vi "main.vi"() -> ()   [LabVIEW 2011]
uses:
  Controls/Open Button.ctl
  Controls/Add2Plot Button.ctl
  Controls/Save Button.ctl
  Controls/Clear Button.ctl
  Controls/Export Button.ctl
  Controls/DAQ Type.ctl
  Controls/Run Button.ctl
  Controls/Stop Button.ctl
  Controls/Progress Bar.ctl
  Controls/Display Mode.ctl
  Controls/User Event Control.ctl
  Controls/User Event Action.ctl
  Controls/User Interface Action.ctl
  Controls/TDMS File Handling.ctl
  Modules/Menu/Menu Action.ctl
  Modules/File/TDMS/TDMS.lvclass
  Functional Global Data/Run Data.ctl
  <vilib>/event_ctls.llb/eventvkey.ctl
  Functional Global Data/Analysis Data.ctl
  Controls/Plot Parameters.ctl
  Functional Global Data/Status Bar.ctl
  Functional Global Data/Globals.ctl
  <vilib>/Utility/error.llb/DialogType.ctl
  Error Handling/Error Module Action.ctl
  <vilib>/Utility/file.llb/Write To Spreadsheet File (DBL).vi
  <vilib>/Analysis/NI_AALBase.lvlib
panel:
  in  "Stop Button":T1
  in  "start DAQ":T2
  in  "Experiment Type":T3
  in  "Open Button":T4
  in  "tab control":enum32{"Data", "Analysis"}(tab)
  in  "Display Mode":T5
  in  "Export History Button":T6
  in  "Run parameters":i32[](listbox)
  in  "Add History 2 Plot Button":T7
  in  "Add Spectrum 2 Plot Button":T7
  out "Notes":string
  out "Run":dbl[][](graph)
  out "Time":i32 caption="Time (s)"
  in  "Sample Channel Number":u32(slide)=1 caption="Sample Number" min=1 max=13 scale=1.0..13.0
  in  "Run Number":u16 caption="Run" min=1 max=1
  out "Sample":cluster{"xo":i32, "dx":i32, dbl[][]}(graph)
  in  "Sample Parameters":i32[](listbox)
  out "Analysis Plot Average":dbl caption="Average"
  in  "Save Concentration Plot Button":T8
  out "Concentration Plot":cluster{dbl[], dbl[]}(graph) caption="concentration VS IMS peak height"
  in  "Clear Plot Button":T9
  in  "Save Plot Button":T8
  out "Analysis Sample Plot":dbl[][](graph)
  out "Progress Bar":T10 scale=0.0..100.0
  out "Status Bar":string="MFC ();"
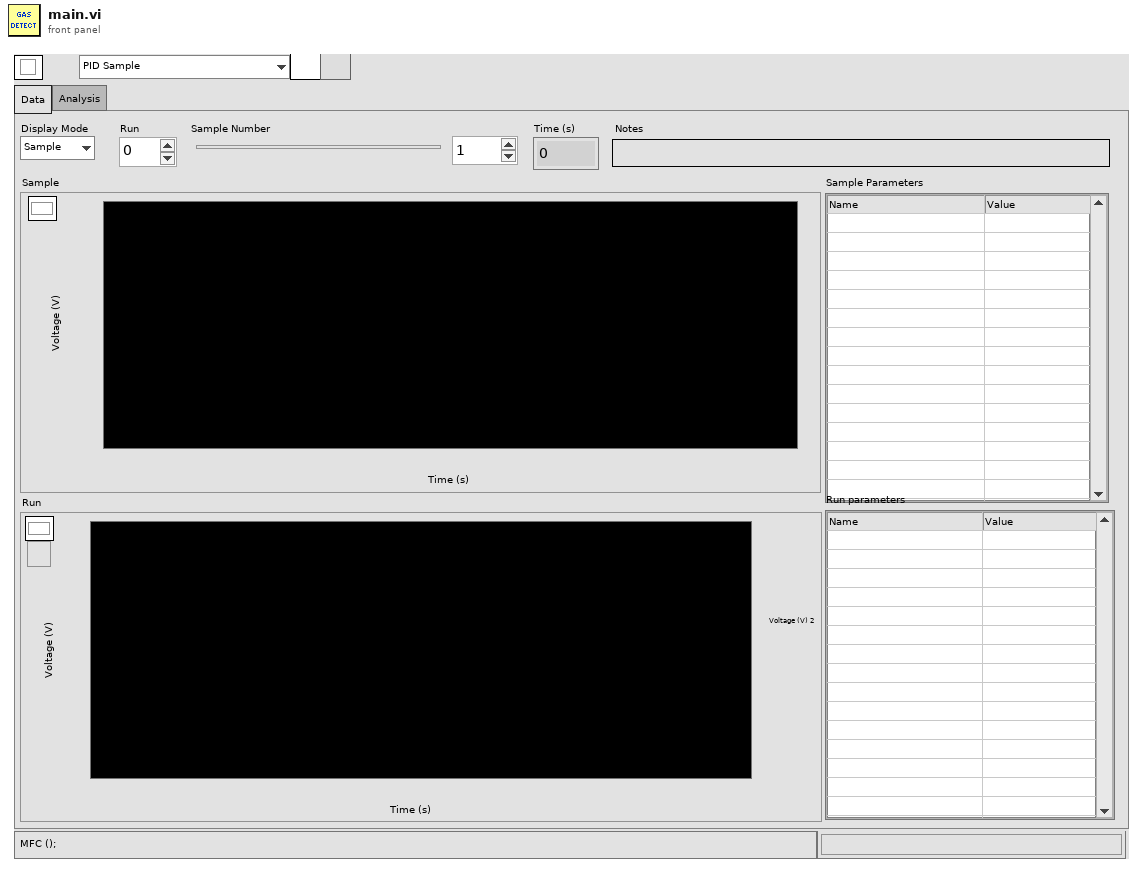
[diagram p1: front panel]
types:
  T1 = typedef "Stop Button.ctl" = bool
  T2 = typedef "Run Button.ctl" = bool
  T3 = typedef "DAQ Type.ctl" = enum16{"PID Sample", "PID with PS Challenge", "PID with MFC Challenge", "Multimeter Sample", "Multimeter with MFC Challenge"}
  T4 = typedef "Open Button.ctl" = bool
  T5 = typedef "Display Mode.ctl" = enum16{"Sample", "Run"}
  T6 = typedef "Export Button.ctl" = bool
  T7 = typedef "Add2Plot Button.ctl" = bool
  T8 = typedef "Save Button.ctl" = bool
  T9 = typedef "Clear Button.ctl" = bool
  T10 = typedef "Progress Bar.ctl" = u8
  T11 = typedef "Class Objects.ctl" = cluster{"configuration":refnum<class "Configuration.lvclass">, "TDMS":refnum<class "TDMS.lvclass">[], "Power Supply":refnum<class "Power Supply.lvclass">, "Mass Flow Controller":refnum<class "Mass Flow Controller.lvclass">, "Valve Controller":refnum<class "Valve Controller.lvclass">, "Multimeter":refnum<class "Multimeter.lvclass">, "Vapour Generator":refnum<class "Vapour Generator.lvclass">, "PIDs":refnum<class "PID.lvclass">[]}
  T12 = typedef "User Event Control.ctl" = cluster{"action":T13, "data":variant}
  T13 = typedef "User Event Action.ctl" = enum16{"Program Initialization", "Device Connections", "Device Settings", "Options", "DAQ Init", "PID Sample Test", "PID with PS Challenge", "PID with MFC Challenge", "Multimeter Sample Test", "Multimeter with MFC Challenge", "DAQ Stop", "Open Data File", "View Data File", "Change Display Mode", "Load INL PID Run Data", "Load Baseline-Mocon PID Data", "Load Multimeter Data", "Set Channel Sample", "Key Down", "Add Spectrum to Plot", "Add History to Plot", "Export History to Excel", "Clear Plots", "Save Plot", "Save Spectral Variable", "History Cursor Release", "Analysis Plot Cursor Release", "Program Deinitialization"}
  T14 = typedef "Menu Action.ctl" = enum16{"Initialize", "Insert Item", "Remove Item", "Set Checked Item", "Get Checked Item", "Get Item Index", "Item Present?", "Stop"}
  T15 = typedef "Globals.ctl" = enum16{"Initialize", "Get DAQ Params", "Get Data Display Params", "Set DAQ Params", "Set Data Display Params"}
  T16 = typedef "User Interface Action.ctl" = enum16{"Initialize", "Data Acquisition Disable", "Data View Disable", "Sample Set", "Sample Set 2D Data", "Sample Set x0 & dx", "Sample Add", "Sample Set Cursor", "Sample Set Offset & Multiplier", "Sample Set Axis Labels", "Sample Parameters Disabled", "Sample Parameters Update", "Run Update", "Run Set Offset & Multiplier", "Run Set Axis Labels", "Run Set Cursor", "Run Set Disabled", "Run Parameters Update", "Run Parameters Disabled", "Run Number Set", "Run Number Set Range", "Run Number Set Disabled", "Sample Number Set", "Sample Number Set Range", "Notes Set Value", "Update Plot", "Set Plot Parameters", "Update Concentration Plot", "Time Set", "Clear DAQ Display", "Clear Analysis Display", "Status Bar Set", "Progress Bar Set", "Display Mode Set", "Experiment Type Set", "Analysis Plot Average Set", "Stop"}
  T17 = typedef "Error Module Action.ctl" = enum16{"Initialize", "Handle Errors", "Report Errors"}
  T18 = typedef "Data Acquisition Parameters.ctl" = cluster{"Experiment Type":T3, "Experiment Name":string, "Operator Name":string, "Notes":string, "TDMS File Path":path, "Data Acquisition State":bool, "PID Voltage Sweep":T19, "MFC Challenge Profile - Heaviside Step":T20, "MFC Challenge Profile":T21, "MFC Challenge Profile - Staircase":T22}
  T19 = typedef "PID Voltage Seep Settings.ctl" = cluster{"Voltage Step (V)":dbl, "Voltage Range (V)":cluster{u16, u16}, "Time Step (s)":dbl, "Voltage Step Direction":enum16{"High 2 Low", "Low 2 High"}}
  T20 = typedef "MFC Challenge Profile - Heaviside Step.ctl" = cluster{"Valve Open Duration":u16, "MFC Flow Rate":dbl, "Valve Open Repeats":u16, "Valve Open Start":u16}
  T21 = typedef "MFC Challen Profile Type.ctl" = enum16{"Heaviside", "Staircase"}
  T22 = typedef "MFC Challenge Profile - Staircase.ctl" = cluster{"Step Time Duration":u16, "Step Flow Rate":dbl, "Steps":u16, "Valve Open Start":u16, "Recovery":bool, "Repeats":u16}
  T23 = typedef "eventvkey.ctl" = enum16{"ASCII", "Enter", "Return", "Shift", "Ctrl", "Alt", "Cmd", "Opt", "Caps", "NumLock", "Clear", "Break", "Up", "Down", "Left", "Right", "Insert", "Delete", "Home", "End", "PageUp", "PageDown", "Escape", "Help", "Pause", "ScrollLock", "F1", "F2", "F3", "F4", "F5", "F6", "F7", "F8", "F9", "F10", "F11", "F12", "F13", "F14", "F15", "F16", "F17", "F18", "F19", "F20", "F21", "F22", "F23", "F24", "Play", "VolumeUp", "VolumeDown", "Mute", "Two Byte Char"}
  T24 = typedef "DialogType.ctl" = u16
  T25 = typedef "TDMS File Handling.ctl" = enum16{"Add TDMS File", "Get Active TDMS File", "Set Active TDMS File", "Set Active TDMS File Index"}
  T26 = typedef "Run Data.ctl" = enum16{"Initialize", "Add Sample Channel", "Set Run", "Get Number of Runs", "Set Run Params", "Get Spectrum", "Get Run Params", "Get Sample Params", "Get History", "Get Averaged History", "Get Run Param Names", "Set Run Param Names", "Get Sample Param Names", "Set Sample Param Names", "Get MFC Flow Rate Challenge Profile", "Get History Average"}
  T27 = typedef "imagedata.ctl" = cluster{"image type":i32, "image depth":i32, "image":u8[], "mask":u8[], "colors":u32[], "Rectangle":cluster{"left":i16, "top":i16, "right":i16, "bottom":i16}}
  T28 = enum8{"Enabled", "Disabled", "Disabled and Grayed Out"}
  T29 = typedef "Analysis Data.ctl" = enum16{"Initialize", "Add Plot", "Get Plots"}
  T30 = typedef "Plot Parameters.ctl" = cluster{"line style":enum16{"0", "1", "2", "3", "4"}, "line width":enum16{"0", "1", "2", "3", "4", "5"}, "plot color":u32}
  T31 = typedef "Status Bar.ctl" = enum16{"Insert Into Status Bar", "Get Status Bar", "Initialize"}
  T32 = enum16{"PID Sample", "PID with PS Challenge", "PID with MFC Challenge", "Multimeter Sample", "Multimeter with MFC Challenge"}
  T33 = typedef "User Interface Control.ctl" = cluster{"action":T16, "data1":variant, "data2":variant}
  T34 = typedef "Challenge.ctl" = cluster{"compound":string, "quantity":dbl, "units":T35, "comment":string}
  T35 = typedef "Concentration Units.ctl" = enum16{"ppt", "ppb", "ppm"}
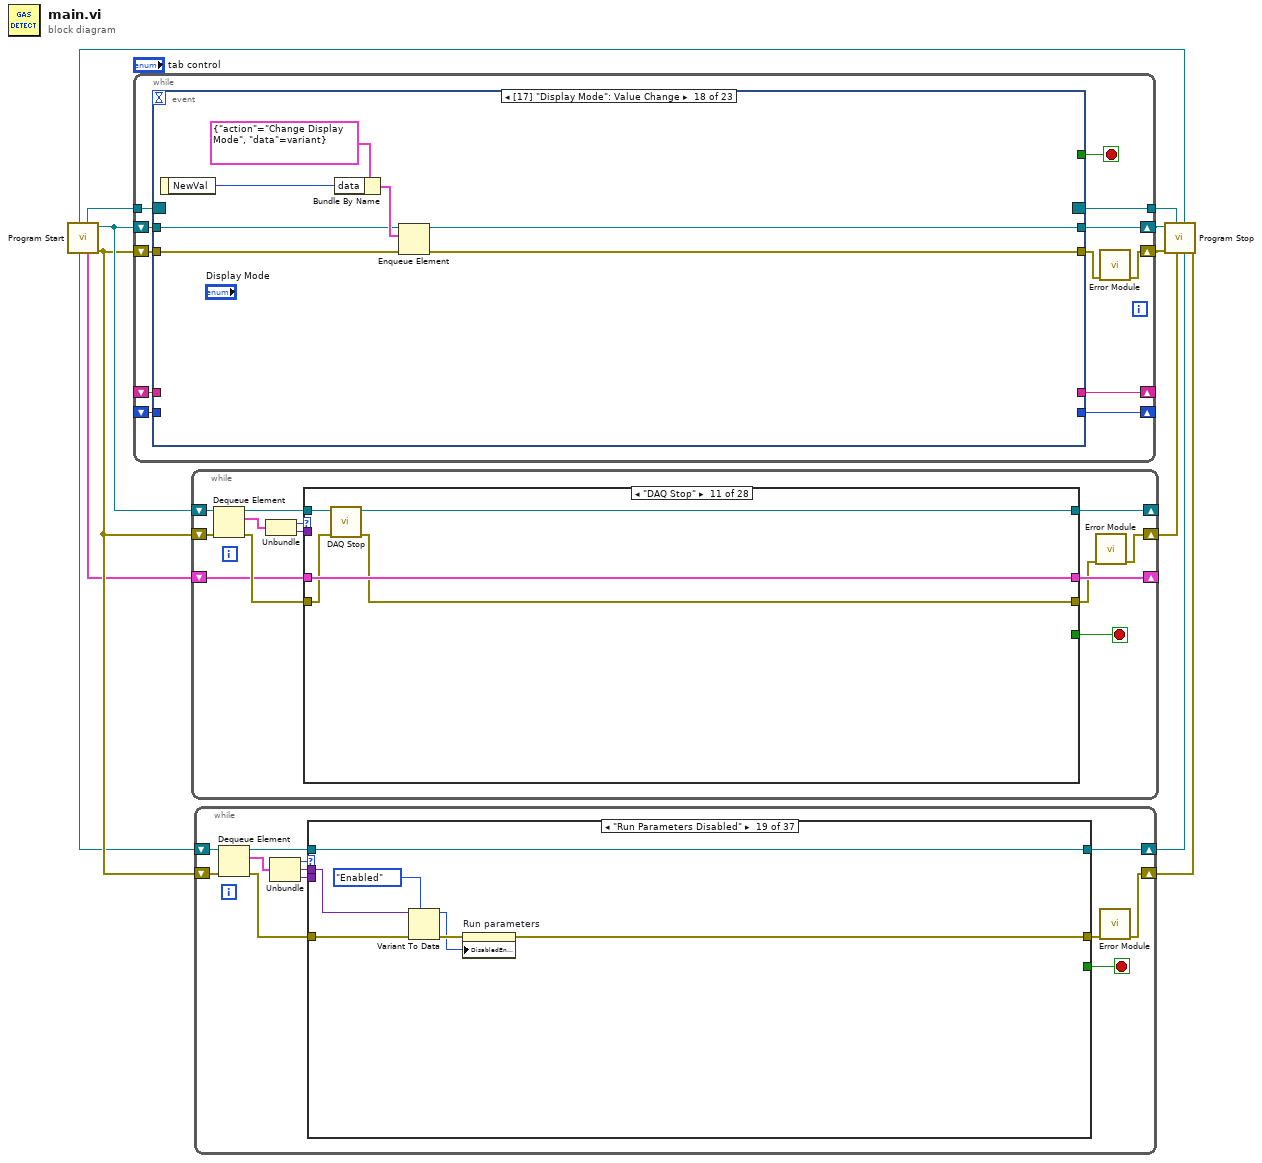
[diagram p0: block diagram]
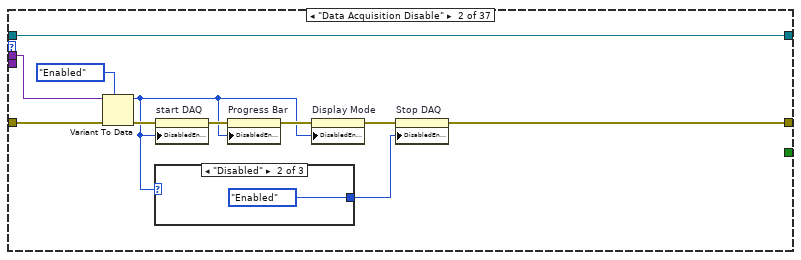
[diagram p3: hidden frame]
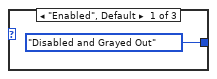
[diagram p4: hidden frame]
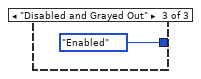
[diagram p5: hidden frame]
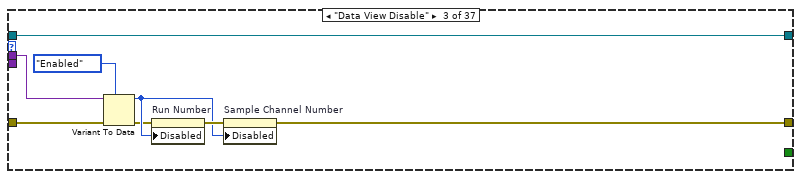
[diagram p6: hidden frame]
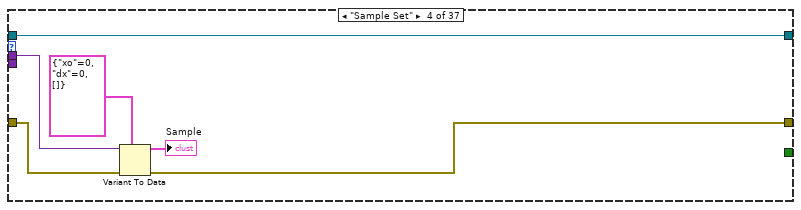
[diagram p7: hidden frame]
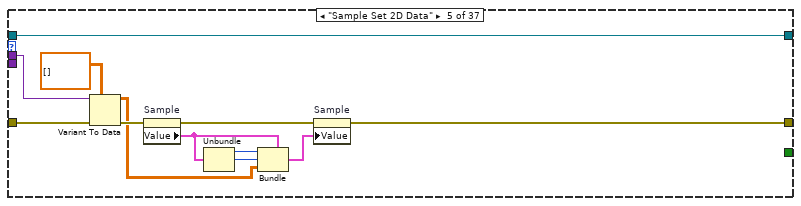
[diagram p8: hidden frame]
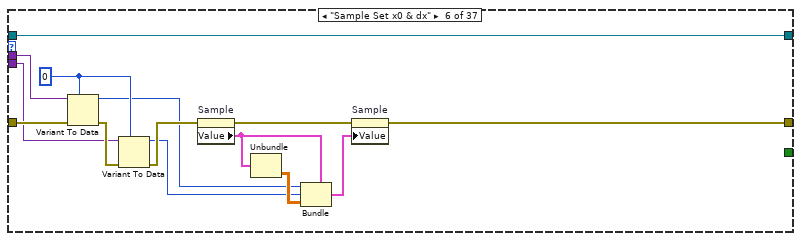
[diagram p9: hidden frame]
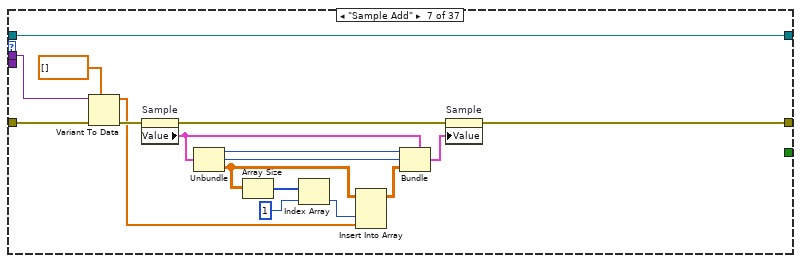
[diagram p10: hidden frame]
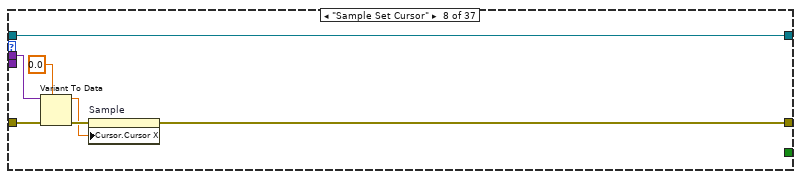
[diagram p11: hidden frame]
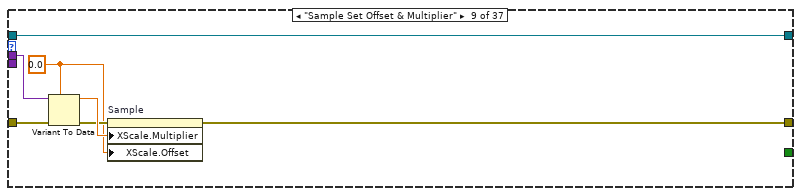
[diagram p12: hidden frame]
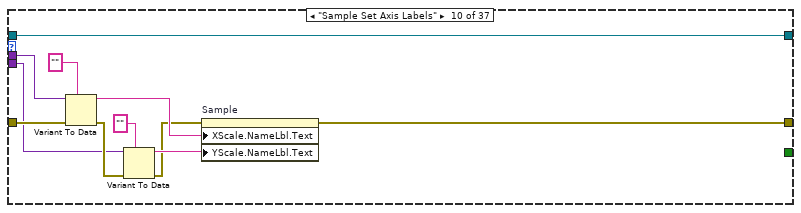
[diagram p13: hidden frame]
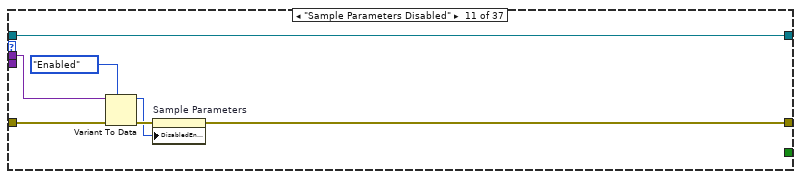
[diagram p14: hidden frame]
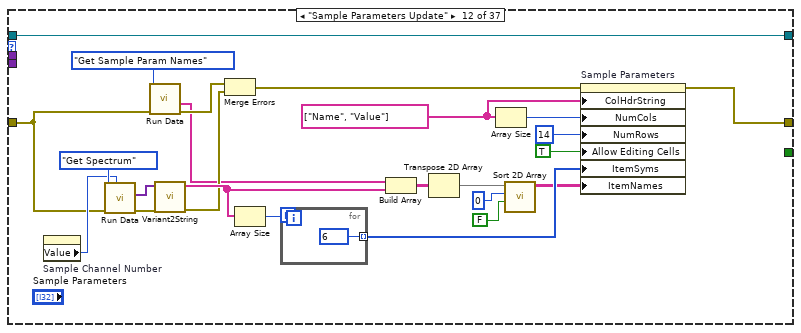
[diagram p15: hidden frame]
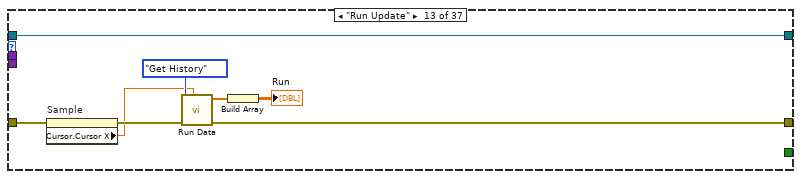
[diagram p16: hidden frame]
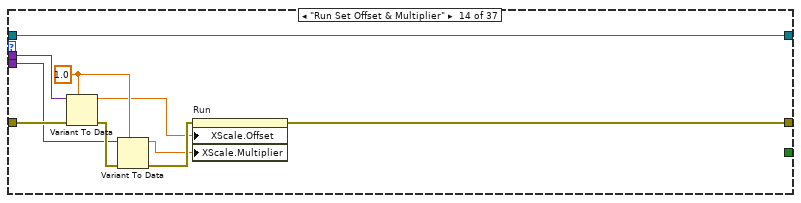
[diagram p17: hidden frame]
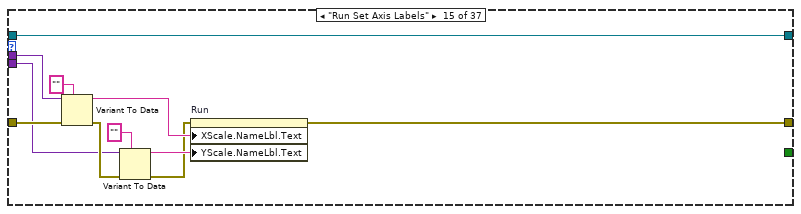
[diagram p18: hidden frame]
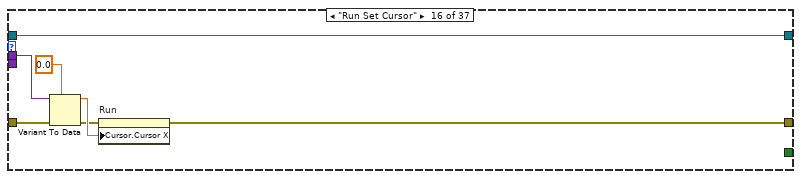
[diagram p19: hidden frame]
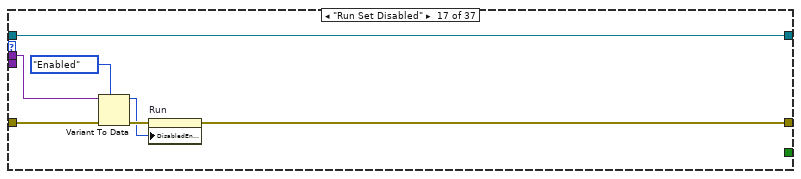
[diagram p20: hidden frame]
diagram:
  n1 = call "Program Start.vi"() -> ("error out"=w10:errorcluster, "user events"=w11:refnum<queue>, "objects"=w6:T11, "Event Registration Refnum out"=w12:refnum<event-registration>, "user interface"=w7:refnum<queue>, "user event"=w8:refnum<user-event>)  [unwired: 6 in]
  n2 = while {
    tunnel: w12 -> [w24]
    tunnel: [w23] -> w9
    shift-right: [w18] -> w5
    shift-left: w11 -> [w21]
    shift-right: [w19] -> w4
    shift-left: w10 -> [w22]
    shift-right: [w16] -> _
    shift-left: _ -> [w15]
    shift-right: [w13] -> _
    shift-left: _ -> [w14]
    stop <- w17 stop-if-true
    n3 = event shown="[17] \"Display Mode\": Value Change" {
      selector: w24 -> [_ _ _ _ _ _ _ _ _ _ _ _ _ _ _ _ _ _ _ _ _ _ _]
      dyn-events: [_ _ _ _ _ _ _ _ _ _ _ _ _ _ _ _ _ _ _ _ _ _ _] -> w23
      timeout: _ -> [_ _ _ _ _ _ _ _ _ _ _ _ _ _ _ _ _ _ _ _ _ _ _]
      tunnel: w22 -> [w29 w155 w163 w183 w190 w193 w199 w203 w208 w213 w218 w223 w226 w232 w242 w248 w263 w272 w282 w286 w294 w330 w339]
      tunnel: [w26 w153 w160 w186 w189 w192 w198 w201 w206 w211 w216 w222 w225 w230 w236 w248 w260 w269 w279 w283 w293 w330 w335] -> w20
      tunnel: w21 -> [w28 w154 w162 w184 w188 w194 w200 w204 w209 w214 w219 w221 w229 w233 w241 w249 w262 w273 w281 w289 w296 w331 w340]
      tunnel: [w27 w154 w161 w187 w188 w191 w197 w202 w207 w212 w217 w221 w228 w231 w240 w249 w259 w270 w280 w284 w295 w331 w340] -> w18
      tunnel: [w25 _ _ _ _ _ _ _ _ _ _ _ _ _ _ _ TRUE _ _ _ _ _ _] -> w17
      tunnel: [_ _ _ _ _ _ _ _ _ _ _ _ _ _ _ _ _ _ _ _ _ w329 _] -> w16
      tunnel: w15 -> [_ _ _ _ _ _ _ _ _ _ _ _ _ _ _ _ _ _ _ _ w297 _ _]
      tunnel: w14 -> [_ _ _ _ _ _ _ _ _ _ _ _ _ _ w235 w245 _ _ _ _ _ _ _]
      tunnel: [_ _ _ _ _ _ _ _ _ _ _ _ _ _ w235 w246 _ _ _ _ _ _ _] -> w13
      event Menu Selection (User) {
        n4 = event-data() -> ("ItemTag"=w30:string)  [unwired: 1 in]
        n5 = case shown="\"Device Connections\"" w30 {
          selector: w30 -> [_ _ _ _ _ w91 _ _ _ _ _ _ _ _ _]
          tunnel: w29 -> [w40 w61 w71 w79 w85 w96 w111 w115 w122 w125 w131 w134 w140 w145 w149]
          tunnel: w28 -> [w33 w63 w73 w80 w88 w95 w110 w116 w120 w126 w128 w137 w141 w146 w150]
          tunnel: [w32 w63 w74 w78 w87 w94 w109 w113 w119 w124 w129 w133 w139 w144 w150] -> w27
          tunnel: [w31 w54 w72 w77 w86 w93 w108 w114 w121 w123 w130 w135 w138 w143 w148] -> w26
          tunnel: [_ _ TRUE _ _ _ _ _ _ _ _ _ _ _ _] -> w25
          frame "Open" {
            n6 = call <vilib>:"Dflt Data Dir.vi"() -> ("App:Default Data Directory"=w41:path)
            n7 = call "File Dialog"("start path"=w41, "error in"=w40, "pattern (all files)"="*.tdms") -> ("selected path"=w34:path, "exists"=w38:bool, "cancelled"=w37:bool, "error out"=w35:errorcluster)  [unwired: 9 in]
            n8 = Compound Arithmetic op=AND(w38, invert w37) -> (w36:bool)
            n9 = case shown="True" w36 {
              tunnel: w34 -> [_ w50]
              tunnel: w35 -> [w44 w52]
              tunnel: [w43 w51] -> w31
              tunnel: w33 -> [w45 w53]
              tunnel: [w45 w46] -> w32
              frame False {
                n10 = call "Clear Specific Error.vi"("error in"=w44, "code"=43 ("Code")) -> ("error out"=w43:errorcluster)  [unwired: 5 in]
              }
              frame True {
                n11 = To Variant(anything=w50) -> (Variant=w48:variant)
                n12 = Bundle By Name(cluster=T12 {"action"=enum."Open Data File", "data"=variant} ("element"), "data"=w48) -> (w47:T12)
                n13 = Enqueue Element(queue=w53, element=w47, error in (no error)=w52) -> (queue out=w46:refnum<queue>, error out=w51:errorcluster)  [unwired: 1 in, 1 out]
              }
            }
          }
          frame "File Viewer" {
            n14 = call <vilib>:"Dflt Data Dir.vi"() -> ("App:Default Data Directory"=w62:path)
            n15 = call "File Dialog2"("start path"=w62, "error in"=w61, "pattern (all files)"="*.tdms") -> ("selected path"=w56:path, "exists"=w59:bool, "cancelled"=w58:bool, "error out"=w55:errorcluster)  [unwired: 9 in]
            n16 = Compound Arithmetic op=AND(w59, invert w58) -> (w57:bool)
            n17 = case shown="False" w57 {
              tunnel: w56 -> [_ w69]
              tunnel: w55 -> [w66 w68]
              tunnel: [w65 w67] -> w54
              frame False {
                n18 = call "Clear Specific Error.vi"("error in"=w66, "code"=43 ("Code")) -> ("error out"=w65:errorcluster)  [unwired: 5 in]
              }
              frame True {
                n19 = call <vilib>:"TDMS - File Viewer.vi"("error in (no error)"=w68, "file path"=w69) -> ("error out"=w67:errorcluster)  [unwired: 4 in, 1 out]
              }
            }
          }
          frame "Exit" {
            w75 = T12 {"action"=enum."Program Deinitialization", "data"=variant}  # user event control
            n20 = call "DAQ Abort.vi"("error in"=w71) -> ("error out"=w70:errorcluster)  [unwired: 9 in]
            n21 = Enqueue Element(queue=w73, element=w75, error in (no error)=w70) -> (queue out=w74:refnum<queue>, error out=w72:errorcluster)  [unwired: 1 in, 1 out]
          }
          frame "DAQ Run" {
            w83 = T12 {"action"=enum."DAQ Init", "data"=variant}  # user event control
            n22 = Bundle By Name(cluster=w83, "data"=FALSE) -> (w81:T12)
            n23 = Enqueue Element(queue=w80, element=w81, error in (no error)=w79) -> (queue out=w78:refnum<queue>, error out=w77:errorcluster)  [unwired: 1 in, 1 out]
          }
          frame "DAQ Stop" {
            w89 = T12 {"action"=enum."DAQ Stop", "data"=variant}  # user event control
            n24 = call "DAQ Abort.vi"("error in"=w85) -> ("error out"=w84:errorcluster)  [unwired: 9 in]
            n25 = Enqueue Element(queue=w88, element=w89, error in (no error)=w84) -> (queue out=w87:refnum<queue>, error out=w86:errorcluster)  [unwired: 1 in, 1 out]
          }
          frame "View", Default {
            n26 = Not Equal?(x=w91, y="View") -> (x != y?=w92:bool)
            n27 = case shown="True" w92 {
              tunnel: w96 -> [w97 w107]
              tunnel: w95 -> [w98 w105]
              tunnel: [w98 w104] -> w94
              tunnel: [w97 w103] -> w93
              tunnel: w91 -> [_ w101]
              frame False {
              }
              frame True {
                n28 = call "Menu.vi"("action"=Menu_Action."Set Checked Item" ("Menu"), "error in"=w107, "item tag"=w101) -> ("error out"=w99:errorcluster)  [unwired: 5 in, 3 out]
                n29 = Bundle By Name(cluster=T12 {"action"=enum."View Data File", "data"=variant} ("element"), "data"=w101) -> (w100:T12)
                n30 = Enqueue Element(queue=w105, element=w100, error in (no error)=w99) -> (queue out=w104:refnum<queue>, error out=w103:errorcluster)  [unwired: 1 in, 1 out]
              }
            }
          }
          frame "Add Spectrum to Plot" {
            n31 = Enqueue Element(queue=w110, element=T12 {"action"=enum."Add Spectrum to Plot", "data"=variant}, error in (no error)=w111) -> (queue out=w109:refnum<queue>, error out=w108:errorcluster)  [unwired: 1 in, 1 out]
          }
          frame "Add History to Plot" {
            n32 = Enqueue Element(queue=w116, element=T12 {"action"=enum."Add History to Plot", "data"=variant}, error in (no error)=w115) -> (queue out=w113:refnum<queue>, error out=w114:errorcluster)  [unwired: 1 in, 1 out]
          }
          frame "Clear Plots" {
            n33 = Enqueue Element(queue=w120, element=T12 {"action"=enum."Clear Plots", "data"=variant}, error in (no error)=w122) -> (queue out=w119:refnum<queue>, error out=w121:errorcluster)  [unwired: 1 in, 1 out]
          }
          frame "Save Plot" {
            n34 = Enqueue Element(queue=w126, element=T12 {"action"=enum."Save Plot", "data"=variant}, error in (no error)=w125) -> (queue out=w124:refnum<queue>, error out=w123:errorcluster)  [unwired: 1 in, 1 out]
          }
          frame "Save Spectral Variable" {
            n35 = Enqueue Element(queue=w128, element=T12 {"action"=enum."Save Spectral Variable", "data"=variant}, error in (no error)=w131) -> (queue out=w129:refnum<queue>, error out=w130:errorcluster)  [unwired: 1 in, 1 out]
          }
          frame "Device Settings" {
            n36 = Enqueue Element(queue=w137, element=T12 {"action"=enum."Device Settings", "data"=variant}, error in (no error)=w134) -> (queue out=w133:refnum<queue>, error out=w135:errorcluster)  [unwired: 1 in, 1 out]
          }
          frame "Device Connections" {
            n37 = Enqueue Element(queue=w141, element=T12 {"action"=enum."Device Connections", "data"=variant}, error in (no error)=w140) -> (queue out=w139:refnum<queue>, error out=w138:errorcluster)  [unwired: 1 in, 1 out]
          }
          frame "Options" {
            n38 = Enqueue Element(queue=w146, element=T12 {"action"=enum."Options", "data"=variant}, error in (no error)=w145) -> (queue out=w144:refnum<queue>, error out=w143:errorcluster)  [unwired: 1 in, 1 out]
          }
          frame "About" {
            n39 = call "About_ANOL.vi"("error in"=w149) -> ("error out"=w148:errorcluster)  [unwired: 10 in]
          }
        }
      }
      event Value Change {
        n40 = event-data() -> ("NewVal"=w152:T3)  [unwired: 1 in]
        n41 = call "Globals.vi"("action"=Globals."Get DAQ Params", "error in"=w155) -> ("error out"=w158:errorcluster, "Data Acquisition"=w157:T18)  [unwired: 7 in, 1 out]
        n42 = Bundle By Name(cluster=w157, "Experiment Type"=w152) -> (w156:T18)
        n43 = call "Globals.vi"("action"=Globals."Set DAQ Params", "error in"=w158, "Data Acquisition"=w156) -> ("error out"=w153:errorcluster)  [unwired: 6 in, 2 out]
      }
      event Value Change {
        n44 = event-data() -> ()  [unwired: 1 in, 1 out]
        n45 = call <vilib>:"Dflt Data Dir.vi"() -> ("App:Default Data Directory"=w170:path)
        n46 = call "File Dialog4"("start path"=w170, "error in"=w163, "pattern (all files)"="*.tdms") -> ("selected path"=w164:path, "exists"=w168:bool, "cancelled"=w167:bool, "error out"=w165:errorcluster)  [unwired: 9 in]
        n47 = Compound Arithmetic op=AND(w168, invert w167) -> (w166:bool)
        n48 = case shown="True" w166 {
          tunnel: w164 -> [_ w179]
          tunnel: w165 -> [w172 w181]
          tunnel: [w171 w180] -> w160
          tunnel: w162 -> [w174 w182]
          tunnel: [w174 w175] -> w161
          frame False {
            n49 = call "Clear Specific Error.vi"("error in"=w172, "code"=43 ("Code")) -> ("error out"=w171:errorcluster)  [unwired: 5 in]
          }
          frame True {
            n50 = To Variant(anything=w179) -> (Variant=w177:variant)
            n51 = Bundle By Name(cluster=T12 {"action"=enum."Open Data File", "data"=variant} ("element"), "data"=w177) -> (w176:T12)
            n52 = Enqueue Element(queue=w182, element=w176, error in (no error)=w181) -> (queue out=w175:refnum<queue>, error out=w180:errorcluster)  [unwired: 1 in, 1 out]
          }
        }
      }
      event Value Change {
        w185 = T12 {"action"=enum."DAQ Init", "data"=variant}  # user event control
        n53 = event-data() -> ()  [unwired: 1 in, 1 out]
        n54 = Enqueue Element(queue=w184, element=w185, error in (no error)=w183) -> (queue out=w187:refnum<queue>, error out=w186:errorcluster)  [unwired: 1 in, 1 out]
      }
      event Value Change {
        n55 = event-data() -> ()  [unwired: 1 in, 1 out]
        n56 = call "DAQ Abort.vi"("error in"=w190) -> ("error out"=w189:errorcluster)  [unwired: 9 in]
      }
      event Value Change {
        n57 = event-data() -> ()  [unwired: 1 in, 1 out]
        n58 = Enqueue Element(queue=w194, element=T12 {"action"=enum."Add Spectrum to Plot", "data"=variant}, error in (no error)=w193) -> (queue out=w191:refnum<queue>, error out=w192:errorcluster)  [unwired: 1 in, 1 out]
      }
      event Value Change {
        n59 = event-data() -> ()  [unwired: 1 in, 1 out]
        n60 = Enqueue Element(queue=w200, element=T12 {"action"=enum."Add History to Plot", "data"=variant}, error in (no error)=w199) -> (queue out=w197:refnum<queue>, error out=w198:errorcluster)  [unwired: 1 in, 1 out]
      }
      event Value Change {
        n61 = event-data() -> ()  [unwired: 1 in, 1 out]
        n62 = Enqueue Element(queue=w204, element=T12 {"action"=enum."Export History to Excel", "data"=variant}, error in (no error)=w203) -> (queue out=w202:refnum<queue>, error out=w201:errorcluster)  [unwired: 1 in, 1 out]
      }
      event Value Change {
        n63 = event-data() -> ()  [unwired: 1 in, 1 out]
        n64 = Enqueue Element(queue=w209, element=T12 {"action"=enum."Save Plot", "data"=variant}, error in (no error)=w208) -> (queue out=w207:refnum<queue>, error out=w206:errorcluster)  [unwired: 1 in, 1 out]
      }
      event Value Change {
        n65 = event-data() -> ()  [unwired: 1 in, 1 out]
        n66 = Enqueue Element(queue=w214, element=T12 {"action"=enum."Clear Plots", "data"=variant}, error in (no error)=w213) -> (queue out=w212:refnum<queue>, error out=w211:errorcluster)  [unwired: 1 in, 1 out]
      }
      event Value Change {
        n67 = event-data() -> ()  [unwired: 1 in, 1 out]
        n68 = Enqueue Element(queue=w219, element=T12 {"action"=enum."Save Spectral Variable", "data"=variant}, error in (no error)=w218) -> (queue out=w217:refnum<queue>, error out=w216:errorcluster)  [unwired: 1 in, 1 out]
      }
      event "Sample": Cursor Release {
        n69 = event-data() -> ()  [unwired: 1 in, 1 out]
        n70 = call "User Interface Global.vi"("error in"=w223, "action"=User_Interface_Action."Run Update" ("Action")) -> ("error out"=w222:errorcluster)  [unwired: 9 in]
      }
      event "Run": Cursor Release {
        n71 = event-data() -> ()  [unwired: 1 in, 1 out]
        n72 = Enqueue Element(queue=w229, element=T12 {"action"=enum."History Cursor Release", "data"=variant}, error in (no error)=w226) -> (queue out=w228:refnum<queue>, error out=w225:errorcluster)  [unwired: 1 in, 1 out]
      }
      event "Analysis Sample Plot": Cursor Release {
        n73 = event-data() -> ()  [unwired: 1 in, 1 out]
        n74 = Enqueue Element(queue=w233, element=T12 {"action"=enum."Analysis Plot Cursor Release", "data"=variant}, error in (no error)=w232) -> (queue out=w231:refnum<queue>, error out=w230:errorcluster)  [unwired: 1 in, 1 out]
      }
      event Key Down; Key Repeat {
        n75 = event-data() -> ("VKey"=w238:T23)  [unwired: 1 in]
        n76 = Bundle By Name(cluster=T12 {"action"=enum."Key Down", "data"=variant} ("element"), "data"=w238) -> (w237:T12)
        n77 = Enqueue Element(queue=w241, element=w237, error in (no error)=w242) -> (queue out=w240:refnum<queue>, error out=w236:errorcluster)  [unwired: 1 in, 1 out]
      }
      event event type 5.0.x8000000b {
        n78 = event-data() -> ("Time"=w244:u32)  [unwired: 1 in]
        n79 = First Call?() -> (First Call?: T/F=w243:bool)
        n80 = case shown="False" w243 {
          tunnel: [w253 TRUE] -> w247
          tunnel: [w252 w257] -> w246
          tunnel: w245 -> [w250 _]
          tunnel: w244 -> [w251 w257]
          frame False {
            n81 = Add(x=w250, y=100) -> (x+y=w254:u32)
            n82 = Less?(x=w251, y=w254) -> (x < y?=w253:bool)
            n83 = Select(t=w250, s=w253, f=w251) -> (s? t:f=w252:u32)
          }
          frame True {
          }
        }
        n84 = event-data("Discard?"=w247) -> ()  [unwired: 1 in, 1 out]
      }
      event Panel Close? {
        w267 = T12 {"action"=enum."Program Deinitialization", "data"=variant}  # user event control
        n85 = event-data() -> ()  [unwired: 1 in, 1 out]
        n86 = call <vilib>:"Stop Timed Structure.vi"("error in (no error)"=w263, "name"="MAIN") -> ("error out"=w264:errorcluster)  [unwired: 9 in]
        n87 = call "Clear Specific Error.vi"("error in"=w264, "code"=-804 ("Code")) -> ("error out"=w261:errorcluster)  [unwired: 5 in]
        n88 = Enqueue Element(queue=w262, element=w267, error in (no error)=w261) -> (queue out=w259:refnum<queue>, error out=w260:errorcluster)  [unwired: 1 in, 1 out]
        n89 = event-data("Discard?"=TRUE) -> ()  [unwired: 1 in, 1 out]
      }
      event Value Change {
        n90 = event-data() -> ("NewVal"=w271:T5)  [unwired: 1 in]
        n91 = Bundle By Name(cluster=T12 {"action"=enum."Change Display Mode", "data"=variant} ("element"), "data"=w271) -> (w274:T12)
        n92 = Enqueue Element(queue=w273, element=w274, error in (no error)=w272) -> (queue out=w270:refnum<queue>, error out=w269:errorcluster)  [unwired: 1 in, 1 out]
      }
      event "Run Number": Value Change {
        n93 = event-data() -> ("NewVal"=w276:u16)  [unwired: 1 in]
        n94 = Bundle By Name(cluster=T12 {"action"=enum."Load INL PID Run Data", "data"=variant} ("element"), "data"=w276) -> (w277:T12)
        n95 = Enqueue Element(queue=w281, element=w277, error in (no error)=w282) -> (queue out=w280:refnum<queue>, error out=w279:errorcluster)  [unwired: 1 in, 1 out]
      }
      event "Sample Channel Number": Value Change {
        n96 = event-data() -> ("NewVal"=w285:u32)  [unwired: 1 in]
        n97 = Bundle By Name(cluster=T12 {"action"=enum."Set Channel Sample", "data"=variant} ("element"), "data"=w285) -> (w287:T12)
        n98 = Enqueue Element(queue=w289, element=w287, error in (no error)=w286) -> (queue out=w284:refnum<queue>, error out=w283:errorcluster)  [unwired: 1 in, 1 out]
      }
      event "Sample Parameters": Edit Cell {
        n99 = event-data() -> ("Coords.Row"=w298:i32, "Coords.Column"=w290:i32)  [unwired: 1 in]
        n100 = Equal?(x=w290, y=1) -> (x = y?=w291:bool)
        n101 = case shown="False" w291 {
          tunnel: w298 -> [w304 w306]
          tunnel: w297 -> [w302 w314]
          tunnel: w296 -> [w300 w312]
          tunnel: [w300 w311] -> w295
          tunnel: w294 -> [w299 w310]
          tunnel: [w299 w309] -> w293
          tunnel: w290 -> [w303 w308]
          frame False {
            n102 = property on="Sample Parameters" class="MCListbox (strict)"() -> ("ItemNames"=w305:string[][])  [unwired: 2 in, 2 out]
            n103 = Replace Array Subset(array=w305, new element=w302, index (row)=w304, index (col)=w303) -> (w301:string[][])
            n104 = property on="Sample Parameters" class="MCListbox (strict)"("ItemNames"=w301) -> ()  [unwired: 2 in, 2 out]
          }
          frame True {
            n105 = property on="Sample Parameters" class="MCListbox (strict)"() -> ("ItemNames"=w315:string[][])  [unwired: 2 in, 2 out]
            n106 = Index Array(array=w315, index (row)=w306, index (col)=w308) -> (element=w307:string)
            n107 = Not Equal?(x=w307, y=w314) -> (x != y?=w313:bool)
            n108 = case shown="True" w313 {
              tunnel: w312 -> [w317 w328]
              tunnel: [w317 w321] -> w311
              tunnel: w310 -> [w316 w324]
              tunnel: [w316 w318] -> w309
              tunnel: w306 -> [_ w325]
              frame False {
              }
              frame True {
                n109 = call "DAQ Abort.vi"("error in"=w324) -> ("error out"=w323:errorcluster)  [unwired: 9 in]
                n110 = Bundle By Name(cluster=T12 {"action"=enum."Add Spectrum to Plot", "data"=variant} ("element"), "data"=w325) -> (w326:T12)
                n111 = Enqueue Element(queue=w328, element=w326, error in (no error)=w323) -> (queue out=w322:refnum<queue>, error out=w319:errorcluster)  [unwired: 1 in, 1 out]
                n112 = Enqueue Element(queue=w322, element=T12 {"action"=enum."PID Sample Test", "data"=variant}, error in (no error)=w319) -> (queue out=w321:refnum<queue>, error out=w318:errorcluster)  [unwired: 1 in, 1 out]
              }
            }
          }
        }
      }
      event "Sample Parameters": Edit Cell? {
        n113 = event-data() -> ("Coords.Row"=w333:i32, "Coords.Column"=w332:i32)  [unwired: 1 in]
        n114 = property on="Sample Parameters" class="MCListbox (strict)"() -> ("ItemNames"=w334:string[][])  [unwired: 2 in, 2 out]
        n115 = Index Array(array=w334, index (row)=w333, index (col)=w332) -> (element=w329:string)
        n116 = event-data() -> ()  [unwired: 3 in, 1 out]
      }
      event User Event {
        w337 = T24 2 items=["no dialog", "OK message", "continue or stop message", "OK message + warnings", "continue/stop + warnings"] ("type of dialog (OK msg:1)")
        n117 = event-data() -> ()  [unwired: 1 in, 1 out]
        n118 = call "Error Module.vi"("Command (Handle Errors"=Error_Module_Action."Report Errors", "error in"=w339) -> ("error out"=w336:errorcluster)  [unwired: 8 in, 1 out]
        n119 = call <vilib>:"General Error Handler.vi"("type of dialog (OK msg:1)"=w337, "error in (no error)"=w336) -> ("error out"=w335:errorcluster)  [unwired: 9 in, 4 out]
      }
    }
    n120 = call "Error Module.vi"("error in"=w20) -> ("error out"=w19:errorcluster)  [unwired: 9 in, 1 out]
  }
  n121 = while {
    shift-right: [w347] -> _
    shift-left: w11 -> [w353]
    shift-right: [w345] -> w3
    shift-left: w10 -> [w352]
    shift-right: [w342] -> _
    shift-left: w6 -> [w343]
    stop <- w346 stop-if-true
    n122 = Dequeue Element(queue=w353, error in (no error)=w352) -> (queue out=w344:refnum<queue>, element=w351:T12, error out=w348:errorcluster)  [unwired: 1 in, 1 out]
    n123 = Unbundle(w351) -> ("action"=w350:T13, "data"=w349:variant)
    n124 = case shown="\"DAQ Stop\"" w350 {
      tunnel: w349 -> [_ _ _ _ _ _ _ _ _ _ _ w441 w465 _ w475 _ _ w508 w518 _ _ _ _ _ _ _ _ _]
      tunnel: w348 -> [w366 w374 w380 w384 w390 w392 w407 w415 w419 w428 w432 w440 w461 w467 w474 w480 w485 w507 w519 w525 w531 w540 w554 w564 w581 w610 w628 w636]
      tunnel: w344 -> [w358 w375 w378 w381 w389 w397 w404 w412 w422 w427 w434 w439 w447 w466 w469 w482 w487 w502 w514 w527 w534 w544 w557 w565 w582 w604 w632 w638]
      tunnel: [w358 w375 w378 w381 w388 w396 w403 w408 w421 w426 w433 w438 w444 w466 w469 w482 w487 w502 w511 w527 w534 w544 w557 w565 w582 w601 w632 w638] -> w347
      tunnel: [w354 w371 w379 w382 w386 w394 w400 w409 w416 w425 w435 w437 w445 w467 w470 w478 w483 w499 w516 w524 w530 w535 w553 w558 w580 w602 w615 w633] -> w341
      tunnel: [_ _ _ _ _ _ _ _ _ _ _ _ _ _ _ _ _ _ _ _ _ _ _ _ _ _ _ TRUE] -> w346
      tunnel: w343 -> [w357 w373 w377 w385 w391 w393 w406 w414 w420 w429 w436 w443 w457 w468 w477 w481 w486 w501 w515 w526 w533 w543 w556 w566 w583 w607 w631 w635]
      tunnel: [w356 w372 w376 w383 w387 w399 w402 w411 w418 w424 w436 w442 w456 w468 w476 w479 w484 w501 w515 w526 w533 w543 w556 w566 w583 w607 w631 w634] -> w342
      frame "Program Initialization", Default {
        w359 = u32 16777238
        n125 = Current VI's Menubar() -> (w365:refnum<k9>)
        n126 = call "Program Initialization.vi"("menu reference"=w365, "error in"=w366, "classes in"=w357) -> ("error out"=w355:errorcluster, "classes out"=w356:T11)  [unwired: 7 in]
        n127 = property on="tab control" class="TabCtl (strict)"(error in=w355, "FG Color"=w359) -> (error out=w363:errorcluster)  [unwired: 1 in, 1 out]
        n128 = property class="VI"(error in=w363) -> (error out=w362:errorcluster, "Panel"=w364:refnum<vi>)  [unwired: 1 in, 1 out]
        n129 = property class="Pnl"(reference=w364, error in=w362) -> (error out=w361:errorcluster, "Panes[]"=w360:refnum<vi>[])  [unwired: 1 out]
        n130 = for {
          tunnel: w360 -> [w369] mode=indexing
          shift-right: [w368] -> w354
          shift-left: w361 -> [w370]
          tunnel: w359 -> [w367]
          n131 = property class="Pane"(reference=w369, error in=w370, "PaneColor"=w367) -> (error out=w368:errorcluster)  [unwired: 1 out]
        }
      }
      frame "Device Connections" {
        n132 = call "Device Connections.vi"("error in"=w374, "Class Objects In"=w373) -> ("error out"=w371:errorcluster, "Class Objects Out"=w372:T11)  [unwired: 8 in]
      }
      frame "Device Settings" {
        n133 = call "Device Settings.vi"("error in"=w380, "Class Objects In"=w377) -> ("error out"=w379:errorcluster, "Class Objects Out"=w376:T11)  [unwired: 8 in]
      }
      frame "Options" {
        n134 = call "Options.vi"("error in"=w384, "class objects in"=w385) -> ("error out"=w382:errorcluster, "class objects out"=w383:T11)  [unwired: 7 in, 1 out]
      }
      frame "DAQ Init" {
        n135 = call "DAQ Initialization.vi"("queue in"=w389, "error in"=w390, "class objects in"=w391) -> ("error out"=w386:errorcluster, "Class objects"=w387:T11, "queue out"=w388:refnum<queue>)  [unwired: 6 in]
      }
      frame "PID Sample Test" {
        n136 = call "PID Sample Test.vi"("error in"=w392, "classes in"=w393) -> ("error out"=w395:errorcluster, "classes out"=w399:T11)  [unwired: 8 in]
        n137 = Enqueue Element(queue=w397, element=T12 {"action"=enum."DAQ Stop", "data"=variant} ("user event control"), error in (no error)=w395) -> (queue out=w396:refnum<queue>, error out=w394:errorcluster)  [unwired: 1 in, 1 out]
      }
      frame "PID with PS Challenge" {
        n138 = call "PID Voltage Sweep.vi"("error in"=w407, "classes in"=w406) -> ("error out"=w401:errorcluster, "classes out"=w402:T11)  [unwired: 8 in]
        n139 = Enqueue Element(queue=w404, element=T12 {"action"=enum."DAQ Stop", "data"=variant} ("user event control"), error in (no error)=w401) -> (queue out=w403:refnum<queue>, error out=w400:errorcluster)  [unwired: 1 in, 1 out]
      }
      frame "PID with MFC Challenge" {
        n140 = call "PID with MFC Challenge.vi"("error in"=w415, "classes in"=w414) -> ("error out"=w410:errorcluster, "classes out"=w411:T11)  [unwired: 8 in]
        n141 = Enqueue Element(queue=w412, element=T12 {"action"=enum."DAQ Stop", "data"=variant} ("user event control"), error in (no error)=w410) -> (queue out=w408:refnum<queue>, error out=w409:errorcluster)  [unwired: 1 in, 1 out]
      }
      frame "Multimeter Sample Test" {
        n142 = call "MM Sample Test.vi"("error in"=w419, "objects IN"=w420) -> ("error out"=w417:errorcluster, "objects OUT"=w418:T11)  [unwired: 8 in]
        n143 = Enqueue Element(queue=w422, element=T12 {"action"=enum."DAQ Stop", "data"=variant} ("user event control"), error in (no error)=w417) -> (queue out=w421:refnum<queue>, error out=w416:errorcluster)  [unwired: 1 in, 1 out]
      }
      frame "Multimeter with MFC Challenge" {
        n144 = call "MM with MFC Challenge.vi"("error in"=w428, "objects IN"=w429) -> ("error out"=w430:errorcluster, "objects OUT"=w424:T11)  [unwired: 8 in]
        n145 = Enqueue Element(queue=w427, element=T12 {"action"=enum."DAQ Stop", "data"=variant} ("user event control"), error in (no error)=w430) -> (queue out=w426:refnum<queue>, error out=w425:errorcluster)  [unwired: 1 in, 1 out]
      }
      frame "DAQ Stop" {
        n146 = call "DAQ Stop.vi"("error in"=w432, "queue in"=w434) -> ("error out"=w435:errorcluster, "queue out"=w433:refnum<queue>)  [unwired: 8 in]
      }
      frame "Open Data File" {
        n147 = call "Open TDMS File.vi"("user event queue in"=w439, "error in"=w440, "file path"=w441, "class objects"=w443) -> ("error out"=w437:errorcluster, "class object"=w442:T11, "user event queue out"=w438:refnum<queue>)  [unwired: 5 in]
      }
      frame "View Data File" {
        n148 = Variant To Data(error in=w461, type="", Variant=w465) -> (data=w463:string, error out=w462:errorcluster)
        n149 = call "Menu.vi"("action"=Menu_Action."Get Item Index" ("Menu"), "error in"=w462, "item tag"=w463) -> ("error out"=w455:errorcluster, "item index"=w459:i32)  [unwired: 5 in, 2 out]
        n150 = call "File Handling.vi"("TDMS File Handling"=TDMS_File_Handling."Set Active TDMS File Index", "error in"=w455, "Active File Index"=w459, "Class objects"=w457) -> ("error out"=w448:errorcluster, "TDMS File"=w449:refnum<class "TDMS.lvclass">, "Class objects"=w456:T11)  [unwired: 5 in]
        n151 = call-dynamic "Read N_Groups.vi"("error in"=w448, "TDMS in"=w449) -> ("error out"=w454:errorcluster, "N_Groups"=w450:u16)  [unwired: 7 in, 1 out]
        n152 = call "User Interface Global.vi"("error in"=w454, "data1"=w450, "action"=User_Interface_Action."Run Number Set") -> ("error out"=w446:errorcluster)  [unwired: 8 in]
        n153 = Bundle By Name(cluster=T12 {"action"=enum."Load INL PID Run Data", "data"=variant} ("element"), "data"=w450) -> (w451:T12)
        n154 = Enqueue Element(queue=w447, element=w451, error in (no error)=w446) -> (queue out=w444:refnum<queue>, error out=w445:errorcluster)  [unwired: 1 in, 1 out]
      }
      frame "Change Display Mode" {
      }
      frame "Load INL PID Run Data" {
        n155 = Variant To Data(error in=w474, type=0, Variant=w475) -> (data=w471:i32, error out=w473:errorcluster)
        n156 = call "Load INL PID Run Data.vi"("error in"=w473, "run number"=w471, "class objects"=w477) -> ("error out"=w470:errorcluster, "class objects"=w476:T11)  [unwired: 7 in]
      }
      frame "Load Baseline-Mocon PID Data" {
        n157 = call "Load Baseline-Mocon PID Data.vi"("error in"=w480, "class objects"=w481) -> ("error out"=w478:errorcluster, "class objects"=w479:T11)  [unwired: 8 in]
      }
      frame "Load Multimeter Data" {
        n158 = call "Load Multimeter Data.vi"("error in"=w485, "class objects"=w486) -> ("error out"=w483:errorcluster, "class objects"=w484:T11)  [unwired: 8 in]
      }
      frame "Set Channel Sample" {
        n159 = Variant To Data(error in=w507, type=0, Variant=w508) -> (data=w497:i32, error out=w505:errorcluster)
        n160 = call "Run Data.vi"("Index Number"=w497, "error in"=w505, "action"=Run_Data."Get Spectrum" ("Action")) -> ("error out"=w504:errorcluster, "Data 1D OUT"=w489:dbl[])  [unwired: 5 in, 2 out]
        n161 = Build Array(w489) -> (w488:dbl[][])
        n162 = call "User Interface Global.vi"("error in"=w504, "data1"=w488, "action"=User_Interface_Action."Sample Set 2D Data" ("Action")) -> ("error out"=w490:errorcluster)  [unwired: 8 in]
        n163 = property on="Run" class="WFGraph (strict)"(error in=w490) -> (error out=w491:errorcluster, "XScale.Multiplier"=w493:dbl, "XScale.Offset"=w496:dbl)  [unwired: 1 in, 1 out]
        n164 = Decrement(x=w497) -> (x-1=w495:i32)
        n165 = Add(x=w496, y=w495) -> (x+y=w494:dbl)
        n166 = Multiply(x=w493, y=w494) -> (x*y=w492:dbl)
        n167 = call "User Interface Global.vi"("error in"=w491, "data1"=w492, "action"=User_Interface_Action."Run Set Cursor") -> ("error out"=w499:errorcluster)  [unwired: 8 in]
      }
      frame "Key Down" {
        n168 = Variant To Data(error in=w519, type=eventvkey."ASCII" ("VKey"), Variant=w518) -> (data=w512:T23, error out=w513:errorcluster)
        n169 = control-ref of="Sample Channel Number"() -> (w510:refnum<vi>)
        n170 = control-ref of="Run Number"() -> (w509:refnum<vi>)
        n171 = call "Key Down.vi"("VKey"=w512, "error in"=w513, "run"=w509, "spectrum number"=w510, "user event \nqueue reference in"=w514) -> ("error out"=w516:errorcluster, "user event\nqueue reference out"=w511:refnum<queue>)  [unwired: 5 in]
      }
      frame "Add Spectrum to Plot" {
        n172 = local read "Sample"() -> (w522:cluster{"xo":i32, "dx":i32, dbl[][]})
        n173 = Unbundle(w522) -> (w521:dbl[][])  [unwired: 2 out]
        n174 = Index Array(array=w521) -> (element=w520:dbl[])  [unwired: 2 in]
        n175 = call "Add2Plot.vi"("error in"=w525, "FP.Title"="Add Spectrum to Plot", "array"=w520) -> ("error out"=w524:errorcluster)  [unwired: 7 in, 1 out]
      }
      frame "Add History to Plot" {
        n176 = local read "Run"() -> (w529:dbl[][])
        n177 = Index Array(array=w529) -> (element=w528:dbl[])  [unwired: 2 in]
        n178 = call "Add2Plot.vi"("error in"=w531, "FP.Title"="Add Yellow History to Plot", "array"=w528) -> ("error out"=w530:errorcluster)  [unwired: 7 in, 1 out]
      }
      frame "Export History to Excel" {
        n179 = call <vilib>:"Dflt Data Dir.vi"() -> ("App:Default Data Directory"=w542:path)
        n180 = call "File Dialog6"("start path"=w542, "prompt"="Select File Name", "error in"=w540, "pattern (all files)"="*.csv") -> ("selected path"=w537:path, "cancelled"=w539:bool, "error out"=w538:errorcluster)  [unwired: 8 in, 1 out]
        n181 = case shown="False" w539 {
          tunnel: w538 -> [w551 w552]
          tunnel: w537 -> [w550 _]
          tunnel: [w548 w552] -> w535
          frame False {
            n182 = property on="Run" class="WFGraph (strict)"(error in=w551) -> (error out=w548:errorcluster, "Value"=w547:dbl[][])  [unwired: 1 in, 1 out]
            n183 = Transpose 2D Array(2D array=w547) -> (transposed array=w545:dbl[][])
            n184 = call-poly <vilib>:"Write To Spreadsheet File.vi"("format (%.3f)"="%.6f", "append to file? (new file:F)"=TRUE, "2D data"=w545, "file path (dialog if empty)"=w550) -> ()  [unwired: 4 in, 1 out]
          }
          frame True {
          }
        }
      }
      frame "Clear Plots" {
        n185 = call "User Interface Global.vi"("error in"=w554, "action"=User_Interface_Action."Clear Analysis Display" ("Action")) -> ("error out"=w553:errorcluster)  [unwired: 9 in]
      }
      frame "Save Plot" {
        n186 = call <vilib>:"Dflt Data Dir.vi"() -> ("App:Default Data Directory"=w562:path)
        n187 = call "File Dialog3"("start path"=w562, "error in"=w564, "pattern (all files)"="*.jpg") -> ("selected path"=w560:path, "cancelled"=w559:bool, "error out"=w561:errorcluster)  [unwired: 9 in, 1 out]
        n188 = case shown="False" w559 {
          tunnel: [w567 w577] -> w558
          tunnel: w561 -> [w575 w578]
          tunnel: w560 -> [w569 _]
          frame False {
            n189 = property on="Analysis Sample Plot" class="WFGraph (strict)"(error in=w575, "Cursor.Visible"=FALSE) -> (error out=w574:errorcluster)  [unwired: 1 in, 1 out]
            n190 = invoke on="Analysis Sample Plot" class="WFGraph (strict)" method="Get Image"(error in=w574, "bg color"=u32 16448250 ("plot color")) -> (error out=w573:errorcluster, "image data"=w570:T27)  [unwired: 4 in, 4 out]
            n191 = property on="Analysis Sample Plot" class="WFGraph (strict)"(error in=w573, "Cursor.Visible"=TRUE) -> (error out=w568:errorcluster)  [unwired: 1 in, 1 out]
            n192 = call <vilib>:"Write JPEG File.vi"("error in (no error)"=w568, "image data"=w570, "path to JPEG file"=w569) -> ("error out"=w567:errorcluster)  [unwired: 7 in, 1 out]
          }
          frame True {
            n193 = call "Clear Specific Error.vi"("error in"=w578, "code"=43 ("Code")) -> ("error out"=w577:errorcluster)  [unwired: 5 in]
          }
        }
      }
      frame "Save Spectral Variable" {
        n194 = call <vilib>:"Dflt Data Dir.vi"() -> ("App:Default Data Directory"=w587:path)
        n195 = call "File Dialog5"("start path"=w587, "error in"=w581, "pattern (all files)"="*.emf") -> ("selected path"=w585:path, "cancelled"=w584:bool, "error out"=w586:errorcluster)  [unwired: 9 in, 1 out]
        n196 = case shown="False" w584 {
          tunnel: [w589 w595] -> w580
          tunnel: w586 -> [w594 w596]
          tunnel: w585 -> [w590 _]
          frame False {
            n197 = invoke on="Concentration Plot" class="XYGraph (strict)" method="Export Image"(error in=w594, "FileType"=enum32{"BMP", "EPS", "EMF", "PICT"}."EMF" ("File Type"), "Target"=enum32{"File", "Clipboard"}."File", "Path"=w590, "HideGrid"=TRUE ("Hide Grid")) -> (error out=w589:errorcluster)  [unwired: 3 in, 7 out]
          }
          frame True {
            n198 = call "Clear Specific Error.vi"("error in"=w596, "code"=43 ("Code")) -> ("error out"=w595:errorcluster)  [unwired: 5 in]
          }
        }
      }
      frame "History Cursor Release" {
        n199 = property on="Run" class="WFGraph (strict)"(error in=w610) -> (error out=w608:errorcluster, "Cursor.Cursor X"=w614:dbl, "XScale.Multiplier"=w611:dbl, "XScale.Offset"=w613:dbl)  [unwired: 1 in, 1 out]
        n200 = Subtract(x=w614, y=w613) -> (x-y=w612:dbl)
        n201 = Divide(x=w612, y=w611) -> (x/y=w606:dbl)
        n202 = Round Toward +Infinity(x=w606) -> (ceil(x): smallest int >= x=w605:dbl)
        n203 = To Long Integer(number=w605) -> (32bit integer=w599:i32)
        n204 = call "User Interface Global.vi"("error in"=w608, "data1"=w599, "action"=User_Interface_Action."Sample Number Set") -> ("error out"=w603:errorcluster)  [unwired: 8 in]
        n205 = Bundle By Name(cluster=T12 {"action"=enum."Set Channel Sample", "data"=variant} ("element"), "data"=w599) -> (w598:T12)
        n206 = Enqueue Element(queue=w604, element=w598, error in (no error)=w603) -> (queue out=w601:refnum<queue>, error out=w602:errorcluster)  [unwired: 1 in, 1 out]
      }
      frame "Analysis Plot Cursor Release" {
        # "Calculate average of data points between two cursors!"
        n207 = property on="Analysis Sample Plot" class="WFGraph (strict)"(error in=w628, "Active Cursor"=u32 0, "Active Cursor"=u32 1) -> (error out=w617:errorcluster, "Cursor.Cursor X"=w627:dbl, "Cursor.Cursor X"=w626:dbl, "Value"=w624:dbl[][])  [unwired: 1 in, 1 out]
        n208 = Build Array(w627, w626) -> (w625:dbl[])
        n209 = Index Array(array=w624) -> (element=w623:dbl[])  [unwired: 2 in]
        n210 = Array Max & Min(array=w625) -> (max value=w622:dbl, min value=w621:dbl)  [unwired: 2 out]
        n211 = Subtract(x=w622, y=w621) -> (x-y=w620:dbl)
        n212 = Array Subset(array=w623, index=w621, length=w620) -> (w619:dbl[])
        n213 = call <vilib>:"Mean.vi"("X"=w619) -> ("mean"=w616:dbl)  [unwired: 1 out]
        n214 = call "User Interface Global.vi"("error in"=w617, "data1"=w616, "action"=User_Interface_Action."Analysis Plot Average Set") -> ("error out"=w615:errorcluster)  [unwired: 8 in]
      }
      frame "Program Deinitialization" {
        n215 = call "Program Deinitialization.vi"("error in"=w636, "classes in"=w635) -> ("error out"=w633:errorcluster, "classes out"=w634:T11)  [unwired: 8 in]
      }
    }
    n216 = call "Error Module.vi"("error in"=w341) -> ("error out"=w345:errorcluster)  [unwired: 9 in, 1 out]
  }
  n217 = while {
    shift-right: [w643] -> w2
    shift-left: w7 -> [w649]
    shift-right: [w640] -> w1
    shift-left: w10 -> [w650]
    stop <- w642 stop-if-true
    n218 = Dequeue Element(queue=w649, error in (no error)=w650) -> (queue out=w644:refnum<queue>, element=w648:T33, error out=w646:errorcluster)  [unwired: 1 in, 1 out]
    n219 = Unbundle(w648) -> ("action"=w647:T16, "data1"=w645:variant, "data2"=w639:variant)
    n220 = case shown="\"Run Parameters Disabled\"" w647 {
      tunnel: w646 -> [w652 w662 w669 w678 w690 w702 w723 w727 w736 w748 w753 w759 w784 w797 w807 w813 w822 w825 w853 w860 w868 w875 w883 w891 w896 w900 w910 w925 w942 w947 w978 w982 w988 w1004 w1017 w1023 w1028]
      tunnel: w645 -> [_ w661 w674 w679 w689 w704 w721 w728 w737 w746 w754 _ _ w798 w805 w814 w821 _ w852 w861 w869 w872 w882 w889 w897 _ w918 _ w941 _ _ _ w984 w1003 w1015 w1024 _]
      tunnel: w644 -> [w651 w663 w673 w680 w691 w703 w722 w730 w732 w738 w755 w779 w788 w795 w806 w812 w823 w846 w851 w855 w867 w874 w878 w886 w895 w907 w908 w923 w938 w960 w974 w983 w987 w1005 w1016 w1020 w1027]
      tunnel: [w651 w663 w673 w680 w691 w703 w722 w730 w732 w738 w755 w779 w788 w795 w806 w812 w823 w846 w851 w855 w867 w874 w878 w886 w895 w907 w908 w923 w938 w960 w974 w983 w987 w1005 w1016 w1020 w1027] -> w643
      tunnel: [w652 w658 w670 w676 w681 w694 w718 w724 w733 w739 w749 w768 w781 w796 w799 w810 w817 w836 w848 w856 w862 w870 w877 w887 w894 w898 w909 w924 w939 w948 w975 w980 w986 w991 w1013 w1021 w1028] -> w641
      tunnel: [_ _ _ _ _ _ _ _ _ _ _ _ _ _ _ _ _ _ _ _ _ _ _ _ _ _ _ _ _ _ _ _ _ _ _ _ TRUE] -> w642
      tunnel: w639 -> [_ _ _ _ _ w693 _ _ _ w740 _ _ _ w793 w803 _ _ _ _ _ _ _ _ _ _ _ w913 _ _ _ _ _ _ _ _ _ _]
      frame "Initialize", Default {
      }
      frame "Data Acquisition Disable" {
        n221 = Variant To Data(error in=w662, type=T28."Enabled" ("Disabled"), Variant=w661) -> (data=w655:T28, error out=w659:errorcluster)
        n222 = case shown="\"Disabled\"" w655 {
          tunnel: [T28."Disabled and Grayed Out" ("Disabled") T28."Enabled" ("Disabled") T28."Enabled" ("Disabled")] -> w654
          frame "Enabled", Default {
          }
          frame "Disabled" {
          }
          frame "Disabled and Grayed Out" {
          }
        }
        n223 = property on="start DAQ" class="Bool"(error in=w659, "DisabledEnum"=w655) -> (error out=w657:errorcluster)  [unwired: 1 in, 1 out]
        n224 = property on="Progress Bar" class="Slide (strict)"(error in=w657, "DisabledEnum"=w655) -> (error out=w656:errorcluster)  [unwired: 1 in, 1 out]
        n225 = property on="Display Mode" class="Enum (strict)"(error in=w656, "DisabledEnum"=w655) -> (error out=w653:errorcluster)  [unwired: 1 in, 1 out]
        n226 = property on="Stop DAQ" class="Bool"(error in=w653, "DisabledEnum"=w654) -> (error out=w658:errorcluster)  [unwired: 1 in, 1 out]
      }
      frame "Data View Disable" {
        n227 = Variant To Data(error in=w669, type=T28."Enabled" ("Disabled"), Variant=w674) -> (data=w671:T28, error out=w668:errorcluster)
        n228 = property on="Run Number" class="DigNum (strict)"(error in=w668, "Disabled"=w671) -> (error out=w672:errorcluster)  [unwired: 1 in, 1 out]
        n229 = property on="Sample Channel Number" class="Slide (strict)"(error in=w672, "Disabled"=w671) -> (error out=w670:errorcluster)  [unwired: 1 in, 1 out]
      }
      frame "Sample Set" {
        n230 = Variant To Data(error in=w678, type=cluster{"xo":i32, "dx":i32, dbl[][]} {"xo"=0, "dx"=0, []} ("output cluster"), Variant=w679) -> (data=→"Sample":cluster{"xo":i32, "dx":i32, dbl[][]}, error out=w676:errorcluster)
      }
      frame "Sample Set 2D Data" {
        n231 = Variant To Data(error in=w690, type=dbl[][] [], Variant=w689) -> (data=w684:dbl[][], error out=w688:errorcluster)
        n232 = property on="Sample" class="WFGraph (strict)"(error in=w688) -> (error out=w687:errorcluster, "Value"=w686:cluster{"xo":i32, "dx":i32, dbl[][]})  [unwired: 1 in, 1 out]
        n233 = Unbundle(w686) -> ("xo"=w685:i32, "dx"=w683:i32)  [unwired: 1 out]
        n234 = Bundle(cluster=w686, "xo"=w685, "dx"=w683, w684) -> (w682:cluster{"xo":i32, "dx":i32, dbl[][]})
        n235 = property on="Sample" class="WFGraph (strict)"(error in=w687, "Value"=w682) -> (error out=w681:errorcluster)  [unwired: 1 in, 1 out]
      }
      frame "Sample Set x0 & dx" {
        w705 = 0
        n236 = Variant To Data(error in=w702, type=w705, Variant=w704) -> (data=w697:i32, error out=w706:errorcluster)
        n237 = Variant To Data(error in=w706, type=w705, Variant=w693) -> (data=w696:i32, error out=w701:errorcluster)
        n238 = property on="Sample" class="WFGraph (strict)"(error in=w701) -> (error out=w700:errorcluster, "Value"=w699:cluster{"xo":i32, "dx":i32, dbl[][]})  [unwired: 1 in, 1 out]
        n239 = Unbundle(w699) -> (w698:dbl[][])  [unwired: 2 out]
        n240 = Bundle(cluster=w699, "xo"=w697, "dx"=w696, w698) -> (w695:cluster{"xo":i32, "dx":i32, dbl[][]})
        n241 = property on="Sample" class="WFGraph (strict)"(error in=w700, "Value"=w695) -> (error out=w694:errorcluster)  [unwired: 1 in, 1 out]
      }
      frame "Sample Add" {
        n242 = Variant To Data(error in=w723, type=dbl[] [], Variant=w721) -> (data=w709:dbl[], error out=w720:errorcluster)
        n243 = property on="Sample" class="WFGraph (strict)"(error in=w720) -> (error out=w719:errorcluster, "Value"=w716:cluster{"xo":i32, "dx":i32, dbl[][]})  [unwired: 1 in, 1 out]
        n244 = Unbundle(w716) -> ("xo"=w714:i32, "dx"=w713:i32, w710:dbl[][])
        n245 = Array Size(array=w710) -> (size(s)=w712:i32[])
        n246 = Index Array(array=w712, index=1) -> (element=w708:i32)
        n247 = Insert Into Array(array=w710, index (col)=w708, new element=w709) -> (w707:dbl[][])  [unwired: 1 in]
        n248 = Bundle(cluster=w716, "xo"=w714, "dx"=w713, w707) -> (w715:cluster{"xo":i32, "dx":i32, dbl[][]})
        n249 = property on="Sample" class="WFGraph (strict)"(error in=w719, "Value"=w715) -> (error out=w718:errorcluster)  [unwired: 1 in, 1 out]
      }
      frame "Sample Set Cursor" {
        n250 = Variant To Data(error in=w727, type=0.0, Variant=w728) -> (data=w725:dbl, error out=w726:errorcluster)
        n251 = property on="Sample" class="WFGraph (strict)"(error in=w726, "Cursor.Cursor X"=w725) -> (error out=w724:errorcluster)  [unwired: 1 in, 1 out]
      }
      frame "Sample Set Offset & Multiplier" {
        w731 = 0.0 ("X Scale.Offset and Multiplier:Multiplier")
        n252 = Variant To Data(error in=w736, type=w731, Variant=w737) -> (data=w735:dbl, error out=w734:errorcluster)
        n253 = property on="Sample" class="WFGraph (strict)"(error in=w734, "XScale.Multiplier"=w735, "XScale.Offset"=w731) -> (error out=w733:errorcluster)  [unwired: 1 in, 1 out]
      }
      frame "Sample Set Axis Labels" {
        n254 = Variant To Data(error in=w748, type="" ("X Scale.Name Label.Text"), Variant=w746) -> (data=w743:string, error out=w744:errorcluster)
        n255 = Variant To Data(error in=w744, type="" ("X Scale.Name Label.Text"), Variant=w740) -> (data=w742:string, error out=w741:errorcluster)
        n256 = property on="Sample" class="WFGraph (strict)"(error in=w741, "XScale.NameLbl.Text"=w743, "YScale.NameLbl.Text"=w742) -> (error out=w739:errorcluster)  [unwired: 1 in, 1 out]
      }
      frame "Sample Parameters Disabled" {
        n257 = Variant To Data(error in=w753, type=T28."Enabled" ("Disabled"), Variant=w754) -> (data=w750:T28, error out=w751:errorcluster)
        n258 = property on="Sample Parameters" class="MCListbox (strict)"(error in=w751, "DisabledEnum"=w750) -> (error out=w749:errorcluster)  [unwired: 1 in, 1 out]
      }
      frame "Sample Parameters Update" {
        w774 = string[] ["Name", "Value"] ("Column Header Strings[]")
        n259 = property on="Sample Channel Number" class="Slide (strict)"() -> ("Value"=w764:u32)  [unwired: 2 in, 2 out]
        n260 = call "Run Data.vi"("Index Number"=w764, "error in"=w759, "action"=Run_Data."Get Spectrum" ("Action")) -> ("error out"=w763:errorcluster, "Params 1D OUT"=w762:variant[])  [unwired: 5 in, 2 out]
        n261 = call "Run Data.vi"("error in"=w759, "action"=Run_Data."Get Sample Param Names") -> ("error out"=w758:errorcluster, "Param Names OUT"=w757:string[])  [unwired: 6 in, 2 out]
        n262 = call "Variant2String.vi"("error in"=w763, "variant array"=w762) -> ("error out"=w761:errorcluster, "string array"=w766:string[])  [unwired: 8 in]
        n263 = Merge Errors(w758, w761) -> (w760:errorcluster)
        n264 = Array Size(array=w766) -> (size(s)=w767:i32)
        n265 = for {
          N: w767 -> [_]
          tunnel: [6] -> w770 mode=indexing
        }
        n266 = Build Array(w757, w766) -> (w775:string[][])
        n267 = Transpose 2D Array(2D array=w775) -> (transposed array=w776:string[][])
        n268 = Array Size(array=w774) -> (size(s)=w773:i32)
        n269 = call "Sort 2D Array.vi"("Sort numerically?"=FALSE ("Sort numerically"), "Column to Sort on"=0, "2D Input Array"=w776) -> ("2D Ouput Array"=w769:string[][])  [unwired: 8 in]
        n270 = property on="Sample Parameters" class="MCListbox (strict)"(error in=w760, "ColHdrString"=w774, "NumCols"=w773, "NumRows"=u32 14 ("Number of Rows"), "Allow Editing Cells"=TRUE, "ItemSyms"=w770, "ItemNames"=w769) -> (error out=w768:errorcluster)  [unwired: 1 in, 1 out]
      }
      frame "Run Update" {
        n271 = property on="Sample" class="WFGraph (strict)"(error in=w784) -> (error out=w783:errorcluster, "Cursor.Cursor X"=w782:dbl)  [unwired: 1 in, 1 out]
        n272 = call "Run Data.vi"("Index Number"=w782, "error in"=w783, "action"=Run_Data."Get History" ("Action")) -> ("error out"=w781:errorcluster, "Data 1D OUT"=w786:dbl[])  [unwired: 5 in, 2 out]
        n273 = Build Array(w786) -> (→"Run":dbl[][])
      }
      frame "Run Set Offset & Multiplier" {
        w791 = 1.0 ("X Scale.Offset and Multiplier:Multiplier")
        n274 = Variant To Data(error in=w797, type=w791, Variant=w798) -> (data=w790:dbl, error out=w794:errorcluster)
        n275 = Variant To Data(error in=w794, type=w791, Variant=w793) -> (data=w789:dbl, error out=w792:errorcluster)
        n276 = property on="Run" class="WFGraph (strict)"(error in=w792, "XScale.Offset"=w790, "XScale.Multiplier"=w789) -> (error out=w796:errorcluster)  [unwired: 1 in, 1 out]
      }
      frame "Run Set Axis Labels" {
        n277 = Variant To Data(error in=w807, type="" ("X Scale.Name Label.Text"), Variant=w805) -> (data=w802:string, error out=w808:errorcluster)
        n278 = Variant To Data(error in=w808, type="" ("X Scale.Name Label.Text"), Variant=w803) -> (data=w801:string, error out=w800:errorcluster)
        n279 = property on="Run" class="WFGraph (strict)"(error in=w800, "XScale.NameLbl.Text"=w802, "YScale.NameLbl.Text"=w801) -> (error out=w799:errorcluster)  [unwired: 1 in, 1 out]
      }
      frame "Run Set Cursor" {
        n280 = Variant To Data(error in=w813, type=0.0, Variant=w814) -> (data=w816:dbl, error out=w811:errorcluster)
        n281 = property on="Run" class="WFGraph (strict)"(error in=w811, "Cursor.Cursor X"=w816) -> (error out=w810:errorcluster)  [unwired: 1 in, 1 out]
      }
      frame "Run Set Disabled" {
        n282 = Variant To Data(error in=w822, type=T28."Enabled" ("Disabled"), Variant=w821) -> (data=w818:T28, error out=w819:errorcluster)
        n283 = property on="Run" class="WFGraph (strict)"(error in=w819, "DisabledEnum"=w818) -> (error out=w817:errorcluster)  [unwired: 1 in, 1 out]
      }
      frame "Run Parameters Update" {
        w838 = string[] ["Name", "Value"] ("Column Header Strings[]")
        n284 = call "Run Data.vi"("error in"=w825, "action"=Run_Data."Get Run Params") -> ("error out"=w831:errorcluster, "Params 1D OUT"=w828:variant[])  [unwired: 6 in, 2 out]
        n285 = call "Run Data.vi"("error in"=w825, "action"=Run_Data."Get Run Param Names") -> ("error out"=w826:errorcluster, "Param Names OUT"=w824:string[])  [unwired: 6 in, 2 out]
        n286 = call "Variant2String.vi"("error in"=w831, "variant array"=w828) -> ("error out"=w829:errorcluster, "string array"=w840:string[])  [unwired: 8 in]
        n287 = Merge Errors(w826, w829) -> (w830:errorcluster)
        n288 = Array Size(array=w840) -> (size(s)=w841:i32)
        n289 = for {
          N: w841 -> [_]
          tunnel: [6] -> w833 mode=indexing
        }
        n290 = Build Array(w824, w840) -> (w842:string[][])
        n291 = Transpose 2D Array(2D array=w842) -> (transposed array=w843:string[][])
        n292 = Array Size(array=w838) -> (size(s)=w839:i32)
        n293 = call "Sort 2D Array.vi"("Sort numerically?"=FALSE ("Sort numerically"), "Column to Sort on"=0, "2D Input Array"=w843) -> ("2D Ouput Array"=w834:string[][])  [unwired: 8 in]
        n294 = property on="Run parameters" class="MCListbox (strict)"(error in=w830, "ColHdrString"=w838, "NumCols"=w839, "NumRows"=u32 14 ("Number of Rows"), "Allow Editing Cells"=TRUE, "ItemSyms"=w833, "ItemNames"=w834) -> (error out=w836:errorcluster)  [unwired: 1 in, 1 out]
      }
      frame "Run Parameters Disabled" {
        n295 = Variant To Data(error in=w853, type=T28."Enabled" ("Disabled"), Variant=w852) -> (data=w849:T28, error out=w850:errorcluster)
        n296 = property on="Run parameters" class="MCListbox (strict)"(error in=w850, "DisabledEnum"=w849) -> (error out=w848:errorcluster)  [unwired: 1 in, 1 out]
      }
      frame "Run Number Set" {
        n297 = Variant To Data(error in=w860, type=u16 0 ("Run"), Variant=w861) -> (data=w858:u16, error out=w857:errorcluster)
        n298 = property on="Run Number" class="DigNum (strict)"(error in=w857, "Value"=w858) -> (error out=w856:errorcluster)  [unwired: 1 in, 1 out]
      }
      frame "Run Number Set Range" {
        n299 = Variant To Data(error in=w868, type=u16 0 ("Run"), Variant=w869) -> (data=w866:u16, error out=w863:errorcluster)
        n300 = property on="Run Number" class="DigNum (strict)"(error in=w863, "Maximum"=w866, "Minimum"=u16 1 ("Run")) -> (error out=w862:errorcluster)  [unwired: 1 in, 1 out]
      }
      frame "Run Number Set Disabled" {
        n301 = Variant To Data(error in=w875, type=T28."Enabled" ("Disabled"), Variant=w872) -> (data=w871:T28, error out=w873:errorcluster)
        n302 = property on="Run Number" class="DigNum (strict)"(error in=w873, "DisabledEnum"=w871) -> (error out=w870:errorcluster)  [unwired: 1 in, 1 out]
      }
      frame "Sample Number Set" {
        n303 = Variant To Data(error in=w883, type=u32 0 ("IMS Spectrum Number"), Variant=w882) -> (data=w879:u32, error out=w880:errorcluster)
        n304 = property on="Sample Channel Number" class="Slide (strict)"(error in=w880, "Value"=w879) -> (error out=w877:errorcluster)  [unwired: 1 in, 1 out]
      }
      frame "Sample Number Set Range" {
        w885 = 1 ("Scale.Range:Minimum")
        n305 = Variant To Data(error in=w891, type=0 ("IMS Spectrum Number"), Variant=w889) -> (data=w884:i32, error out=w888:errorcluster)
        n306 = property on="Sample Channel Number" class="Slide (strict)"(error in=w888, "Scale.Minimum"=w885, "Minimum"=w885, "Scale.Maximum"=w884, "Maximum"=w884) -> (error out=w887:errorcluster)  [unwired: 1 in, 1 out]
      }
      frame "Notes Set Value" {
        n307 = Variant To Data(error in=w896, type="" ("Notes"), Variant=w897) -> (data=→"Notes":string, error out=w894:errorcluster)
      }
      frame "Update Plot" {
        n308 = call "Analysis Plots.vi"("action"=Analysis_Data."Get Plots" ("Action"), "error in"=w900) -> ("error out"=w899:errorcluster, "plots"=w901:dbl[][])  [unwired: 7 in, 1 out]
        "Analysis Sample Plot" <- w901
        n309 = Array Size(array=w901) -> (size(s)=w906:i32[])
        n310 = Index Array(array=w906) -> (element=w904:i32)  [unwired: 1 in]
        n311 = property on="Analysis Sample Plot" class="WFGraph (strict)"(error in=w899, "LegNumRows"=w904) -> (error out=w905:errorcluster)  [unwired: 1 in, 1 out]
        n312 = Decrement(x=w904) -> (x-1=w903:i32)
        n313 = property on="Analysis Sample Plot" class="WFGraph (strict)"(error in=w905, "Active Plot"=w903) -> (error out=w898:errorcluster)  [unwired: 1 in, 1 out]
      }
      frame "Set Plot Parameters" {
        n314 = Variant To Data(error in=w910, type="" ("Plot.Plot Name"), Variant=w918) -> (data=w915:string, error out=w914:errorcluster)
        n315 = Variant To Data(error in=w914, type=T30 {"line style"=enum."0", "line width"=enum."0", "plot color"=0} ("plot parameters"), Variant=w913) -> (data=w912:T30, error out=w911:errorcluster)
        n316 = Unbundle By Name(w912) -> ("line style"=w922:enum16{"0", "1", "2", "3", "4"}, "line width"=w921:enum16{"0", "1", "2", "3", "4", "5"}, "plot color"=w920:u32)
        n317 = property on="Analysis Sample Plot" class="WFGraph (strict)"(error in=w911, "Plot.Plot Name"=w915, "LegAutosize"=TRUE ("Legend:Autosize"), "Plot.Line Style"=w922, "Plot.Line Width"=w921, "Plot.Plot Color"=w920) -> (error out=w909:errorcluster)  [unwired: 1 in, 1 out]
      }
      frame "Update Concentration Plot" {
        n318 = call "Analysis Plots.vi"("action"=Analysis_Data."Get Plots", "error in"=w925) -> ("error out"=w924:errorcluster, "challenges"=w930:T34[], "plots"=w929:dbl[][])  [unwired: 7 in]
        n319 = for {
          tunnel: w930 -> [w936] mode=indexing
          tunnel: [w935] -> w928 mode=indexing
          tunnel: w929 -> [w933] mode=indexing
          tunnel: [w932] -> w927 mode=indexing
          n320 = Unbundle By Name(w936) -> ("quantity"=w935:dbl)
          n321 = property on="Analysis Sample Plot" class="WFGraph (strict)"() -> ("Cursor.Cursor X"=w934:dbl)  [unwired: 2 in, 2 out]
          n322 = Index Array(array=w933, index=w934) -> (element=w932:dbl)
        }
        n323 = Bundle(w928, w927) -> (→"Concentration Plot":cluster{dbl[], dbl[]})  [unwired: 1 in]
      }
      frame "Time Set" {
        n324 = Variant To Data(error in=w942, type=0 ("IMS Spectrum Number"), Variant=w941) -> (data=→"Time":i32, error out=w939:errorcluster)
      }
      frame "Clear DAQ Display" {
        w950 = string[][] [] ("Item Names")
        w958 = 0 ("Time (s)")
        w959 = 1 ("Time (s)")
        n325 = Index Array(array=dbl[][] []) -> (element=w946:dbl[])  [unwired: 2 in]
        n326 = local write "Sample"(cluster{"xo":i32, "dx":i32, dbl[][]} {"xo"=0, "dx"=0, []} ("output cluster")) -> ()
        n327 = property on="Sample Channel Number" class="Slide (strict)"(error in=w947, "Maximum"=w959, "Scale.Maximum"=w959, "Scale.Minimum"=w958, "Minimum"=w958) -> (error out=w948:errorcluster)  [unwired: 1 in, 1 out]
        n328 = Bundle(w946, w946) -> (w945:cluster{dbl[], dbl[]})  [unwired: 1 in]
        n329 = local write "Concentration Plot"(w945) -> ()
        n330 = local write "Run"(dbl[][] [] ("Plot")) -> ()
        n331 = for {
          N: 10 -> [_]
          i -> [w966]
          n332 = Increment(x=w966) -> (x+1=w962:i32)
          n333 = Number To Decimal String(number=w962) -> (decimal integer string=w963:string)  [unwired: 1 in]
          n334 = Concatenate Strings("Plot " ("string"), w963) -> (w965:string)
          n335 = property on="Analysis Sample Plot" class="WFGraph (strict)"("Active Plot"=w962, "Plot.Plot Name"=w965, "LegAutosize"=TRUE ("Legend:Autosize")) -> ()  [unwired: 2 in, 2 out]
        }
        n336 = property on="Sample Parameters" class="MCListbox (strict)"("ItemNames"=w950) -> ()  [unwired: 2 in, 2 out]
        n337 = property on="Run parameters" class="MCListbox (strict)"("ItemNames"=w950) -> ()  [unwired: 2 in, 2 out]
        n338 = property on="Analysis Sample Plot" class="WFGraph (strict)"("LegNumRows"=u32 1 ("Legend:Number of Rows"), "Active Plot"=u32 0, "Plot.Plot Name"="plot name", "Plot.Line Width"=u8 0, "Plot.Plot Color"=u32 0 ("Plot Color"), "LegAutosize"=FALSE ("Legend:Autosize")) -> ()  [unwired: 2 in, 2 out]
      }
      frame "Clear Analysis Display" {
        w968 = dbl[] []
        n339 = call "Analysis Plots.vi"("action"=Analysis_Data."Initialize" ("Action"), "error in"=w978) -> ("error out"=w975:errorcluster, "plots"=w976:dbl[][])  [unwired: 7 in, 1 out]
        n340 = local write "Analysis Sample Plot"(w976) -> ()
        n341 = Bundle(w968, w968) -> (w967:cluster{dbl[], dbl[]})  [unwired: 1 in]
        n342 = property on="Analysis Sample Plot" class="WFGraph (strict)"("LegNumRows"=u32 1 ("Legend:Number of Rows"), "Active Plot"=u32 0, "Plot.Plot Name"="plot name", "Plot.Line Width"=u8 0, "Plot.Plot Color"=u32 0 ("Plot Color")) -> ()  [unwired: 2 in, 2 out]
        n343 = local write "Concentration Plot"(w967) -> ()
      }
      frame "Status Bar Set" {
        n344 = call "Status Bar.vi"("action"=Status_Bar."Get Status Bar", "error in"=w982) -> ("error out"=w980:errorcluster, "Status Bar"=→"Status Bar":string)  [unwired: 8 in]
      }
      frame "Progress Bar Set" {
        n345 = Variant To Data(error in=w988, type=u8 0 ("IMS Spectrum Number"), Variant=w984) -> (data=→"Progress Bar":u8, error out=w986:errorcluster)
      }
      frame "Display Mode Set" {
        # "Problem when closing application...\nExucute in situ instead!"
        n346 = Variant To Data(error in=w1004, type=Display_Mode."Sample" ("Display Mode 2"), Variant=w1003) -> (data=w1000:T5, error out=w1002:errorcluster)
        n347 = property on="Display Mode" class="Enum (strict)"(error in=w1002, "Value"=w1000) -> (error out=w999:errorcluster)  [unwired: 1 in, 1 out]
        n348 = case shown="\"Run\"" w1000 {
          tunnel: w999 -> [w1007 w1010]
          tunnel: [T28."Enabled" ("Disabled") T28."Disabled and Grayed Out" ("Disabled")] -> w990
          tunnel: [w1007 w1008] -> w993
          frame "Sample", Default {
          }
          frame "Run" {
            n349 = call "User Interface Global.vi"("error in"=w1010, "data1"=1, "action"=User_Interface_Action."Run Number Set") -> ("error out"=w1008:errorcluster)  [unwired: 8 in]
          }
        }
        n350 = call "User Interface Global.vi"("error in"=w993, "data1"=w990, "action"=User_Interface_Action."Run Number Set Disabled") -> ("error out"=w996:errorcluster)  [unwired: 8 in]
        n351 = call "User Interface Global.vi"("error in"=w996, "data1"=w990, "action"=User_Interface_Action."Run Parameters Disabled") -> ("error out"=w994:errorcluster)  [unwired: 8 in]
        n352 = call "User Interface Global.vi"("error in"=w996, "data1"=w990, "action"=User_Interface_Action."Run Set Disabled") -> ("error out"=w995:errorcluster)  [unwired: 8 in]
        n353 = Merge Errors(w995, w994) -> (w991:errorcluster)
      }
      frame "Experiment Type Set" {
        n354 = Variant To Data(error in=w1017, type=T32."Multimeter Sample", Variant=w1015) -> (data=w1014:T32, error out=w1018:errorcluster)
        n355 = property on="Experiment Type" class="Enum (strict)"(error in=w1018, "Value"=w1014) -> (error out=w1013:errorcluster)  [unwired: 1 in, 1 out]
      }
      frame "Analysis Plot Average Set" {
        n356 = Variant To Data(error in=w1023, type=0.0 ("IMS Spectrum Number"), Variant=w1024) -> (data=→"Analysis Plot Average":dbl, error out=w1021:errorcluster)
      }
      frame "Stop" {
      }
    }
    n357 = call "Error Module.vi"("error in"=w641) -> ("error out"=w640:errorcluster)  [unwired: 9 in, 1 out]
  }
  n358 = call "Program Stop.vi"("GUI error"=w1, "user interface"=w2, "user event"=w8, "operation error"=w3, "Event Registration Refnum"=w9, "FP control error"=w4, "user events"=w5) -> ()  [unwired: 5 in]
